vi "Universial XsYa plot.vi"() -> ()   [LabVIEW 2021]
panel:
  in  "Book number":i32=683
  in  "parent data folder":path=path "C:/Users/gyue/Box/Guang Yue uiuc research box folder/data/Contour plot"
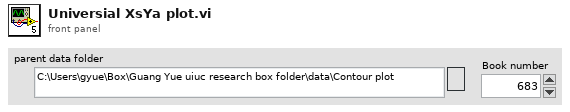
[diagram p1: front panel]
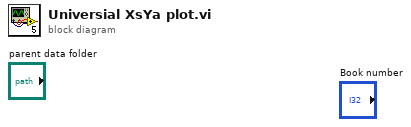
[diagram p0: block diagram]
diagram:
